vi "close.vi"(8 "error in (no error)":errorcluster, 11 "Database.lvclass":refnum<class "Database.lvclass">) -> (0 "error out":errorcluster)   [LabVIEW 2018, in "Database.lvclass"]
uses:
  Database.lvclass
  Database.lvclass/Database.ctl
  <vilib>/addons/database/NI_Database_API.lvlib
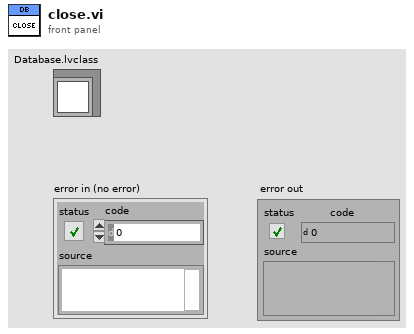
[diagram p1: front panel]
types:
  T1 = typedef "NI_Database_API.lvlib/Conn ObjectReference.ctl" = refnum<k1>
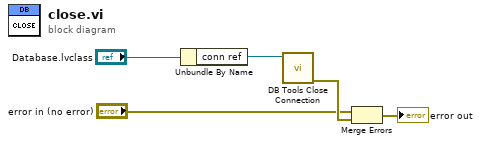
[diagram p0: block diagram]
diagram:
  n1 = Unbundle By Name("Database.lvclass") -> ("conn ref"=w4:T1)
  n2 = call <vilib>:"DB Tools Close Connection.vi"("connection reference"=w4) -> ("error out"=w3:errorcluster)  [unwired: 6 in]
  n3 = Merge Errors("error in (no error)", w3) -> (→"error out":errorcluster)
